vi "Frame Switch by Num.vi"(8 "error in (no error)":errorcluster, 10 "Frame Num":u32, 11 "LF2R IDE in":refnum<class "Main Panel.lvclass">) -> (0 "error out":errorcluster, 3 "LF2R IDE out":refnum<class "Main Panel.lvclass">)   [LabVIEW 2018, in "Main Panel.lvlib" / "Main Panel.lvclass"]
uses:
  Main Panel.lvclass
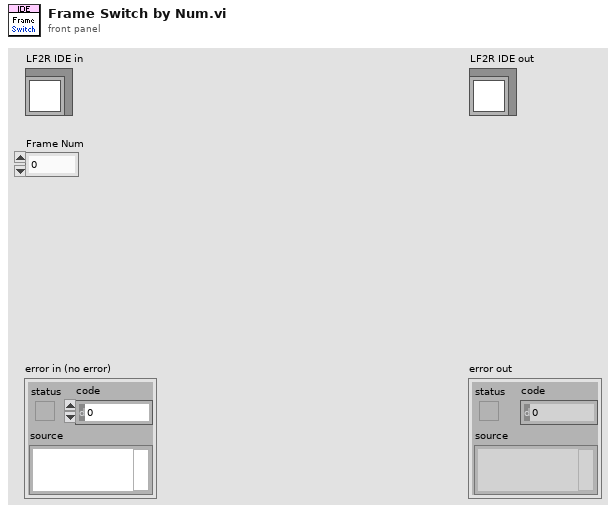
[diagram p1: front panel]
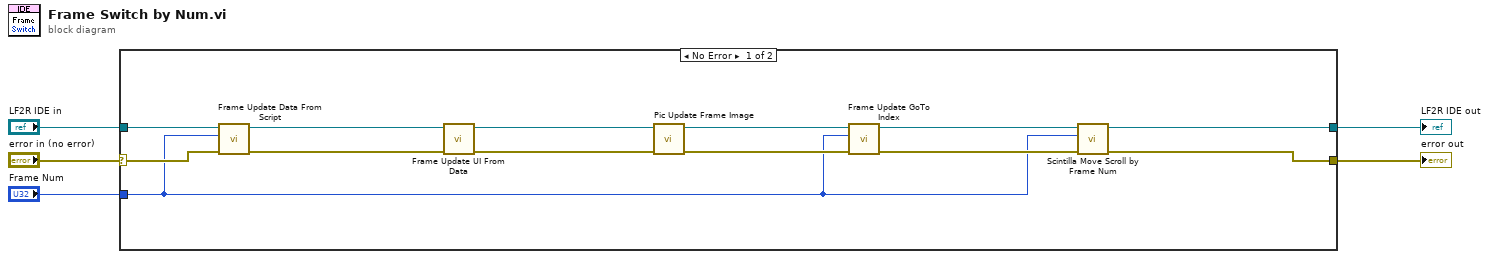
[diagram p0: block diagram]
diagram:
  n1 = case shown="No Error" "error in (no error)" {
    selector: "error in (no error)" -> [w15 w20]
    tunnel: [w13 w20] -> w3
    tunnel: [w14 w19] -> w4
    tunnel: "LF2R IDE in" -> [w18 w19]
    tunnel: "Frame Num" -> [w6 _]
    frame No Error {
      n2 = call "Frame Update Data From Script.vi"("error in (no error)"=w15, "Frame Number"=w6, "IDE simple in"=w18) -> ("error out"=w16:errorcluster, "IDE simple out"=w17:refnum<class "Main Panel.lvclass">)  [unwired: 7 in]
      n3 = call "Frame Update UI From Data.vi"("error in (no error)"=w16, "IDE simple in"=w17) -> ("error out"=w11:errorcluster, "IDE simple out"=w12:refnum<class "Main Panel.lvclass">)  [unwired: 8 in]
      n4 = call "Pic Update Frame Image.vi"("error in (no error)"=w11, "LF2R IDE in"=w12) -> ("error out"=w9:errorcluster, "LF2R IDE out"=w10:refnum<class "Main Panel.lvclass">)  [unwired: 8 in]
      n5 = call "Frame Update GoTo Index.vi"("error in (no error)"=w9, "Frame Num"=w6, "LF2R IDE in"=w10) -> ("error out"=w7:errorcluster, "LF2R IDE out"=w8:refnum<class "Main Panel.lvclass">)  [unwired: 7 in]
      n6 = call "Scintilla Move Scroll by Frame Num.vi"("error in (no error)"=w7, "Frame Number"=w6, "IDE simple in"=w8) -> ("error out"=w13:errorcluster, "IDE simple out"=w14:refnum<class "Main Panel.lvclass">)  [unwired: 7 in]
    }
    frame Error {
    }
  }
  "error out" <- w3
  "LF2R IDE out" <- w4
